vi "Msg EnQ.vi"(5 "Data":variant, 7 "Module Action":T1, 8 "error in (no error)":errorcluster) -> (0 "error out":errorcluster)   [LabVIEW 2021, in "Config Database.lvlib"]
uses:
  Config Database.lvlib
  Private Controls/Module Action.ctl
  Private Controls/Q Control.ctl
  Private Controls/Q Msg Dataset.ctl
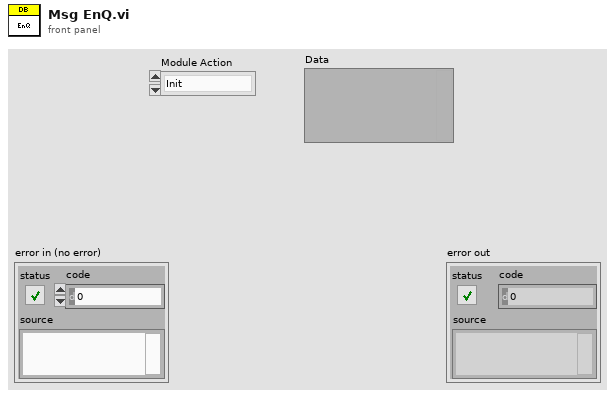
[diagram p1: front panel]
types:
  T1 = typedef "Config Database.lvlib/Module Action.ctl" = enum16{"Init", "Error", "Close", "PreUUT", "Test Execution", "PostUUT"}
  T2 = typedef "Config Database.lvlib/Q Msg Dataset.ctl" = cluster{"Module Action":T1, "Data":variant}
  T3 = typedef "Config Database.lvlib/Q Control.ctl" = enum16{"Obtain", "Get", "Release"}
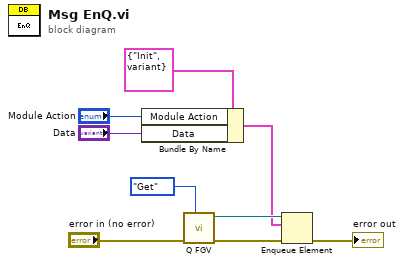
[diagram p0: block diagram]
diagram:
  n1 = Bundle By Name(cluster=T2 {"Module Action"=enum."Init", "Data"=variant} ("Q Msg Dataset"), "Module Action"="Module Action", "Data"="Data") -> (w3:T2)
  n2 = call "Q FGV.vi"("Q Control"=Q_Control."Get", "error in (no error)"="error in (no error)") -> ("error out"=w7:errorcluster, "queue out"=w5:refnum<queue>)  [unwired: 8 in]
  n3 = Enqueue Element(queue=w5, element=w3, error in (no error)=w7) -> (error out=→"error out":errorcluster)  [unwired: 1 in, 2 out]
